vi "retrieveErrorOutput.vi"(8 "error in (no error)":errorcluster, 11 "VI in":refnum<vi>) -> (0 "error out":errorcluster, 1 "VI Error Out":errorcluster, 3 "VI out":refnum<vi>)   [LabVIEW 2013, in "openCronJob.lvlib" / "Job.StaticVIRef.lvclass"]
uses:
  Job.StaticVIRef.lvclass
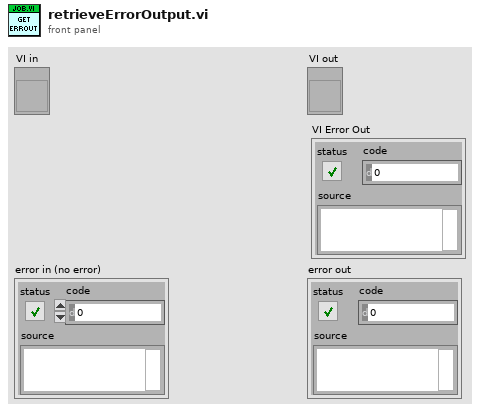
[diagram p1: front panel]
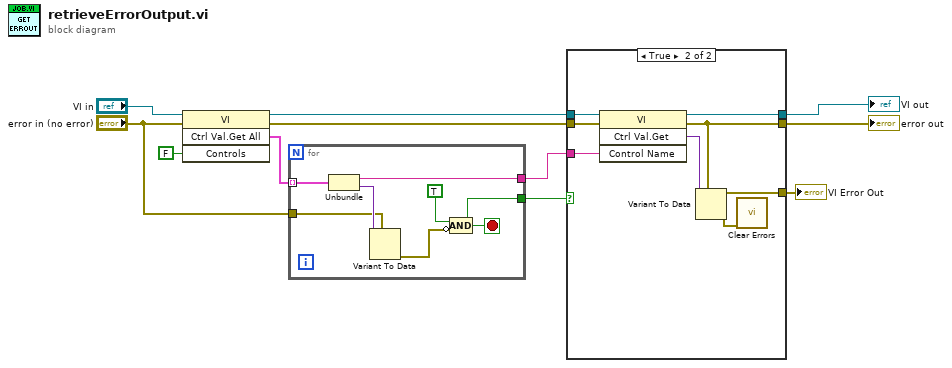
[diagram p0: block diagram]
diagram:
  n1 = invoke class="VI" method="Ctrl Val.Get All"(reference="VI in", error in="error in (no error)", "Controls"=FALSE) -> (reference out=w7:refnum<vi>, error out=w6:errorcluster, "Get All Control Values Variant"=w5:cluster{"Name":string, "Variant Data":variant}[])  [unwired: 1 in, 1 out]
  n2 = for {
    tunnel: w5 -> [w18] mode=indexing
    tunnel: "error in (no error)" -> [w16]
    tunnel: [w14] -> w4
    tunnel: [w12] -> w1
    stop <- w14 stop-if-true
    n3 = Unbundle(w18) -> ("Name"=w12:string, "Variant Data"=w17:variant)
    n4 = Variant To Data(type=w16, Variant=w17) -> (error out=w15:errorcluster)  [unwired: 1 in, 1 out]
    n5 = Compound Arithmetic op=AND(TRUE, invert w15) -> (w14:bool)
  }
  n6 = case shown="True" w4 {
    tunnel: [w19 w22] -> w11
    tunnel: [w20 w28] -> w10
    tunnel: w7 -> [w20 w27]
    tunnel: w6 -> [w19 w26]
    tunnel: [_ w24] -> w2
    tunnel: w1 -> [_ w21]
    frame False {
    }
    frame True {
      n7 = invoke class="VI" method="Ctrl Val.Get"(reference=w27, error in=w26, "Control Name"=w21) -> (reference out=w28:refnum<vi>, error out=w22:errorcluster, "Get Control Value Variant"=w25:variant)  [unwired: 1 in, 1 out]
      n8 = Variant To Data(type=w22, Variant=w25) -> (data=w24:errorcluster, error out=w23:errorcluster)  [unwired: 1 in]
      n9 = call <vilib>:"Clear Errors.vi"("error in (no error)"=w23) -> ()  [unwired: 6 in, 1 out]
    }
  }
  "error out" <- w11
  "VI out" <- w10
  "VI Error Out" <- w2
